vi "Voltage_Sweep_pts.vi"(9 "Vref_Voltage":dbl, 11 "Points":i32) -> (2 "Array":dbl[](array[numeric]))   [LabVIEW 2019]
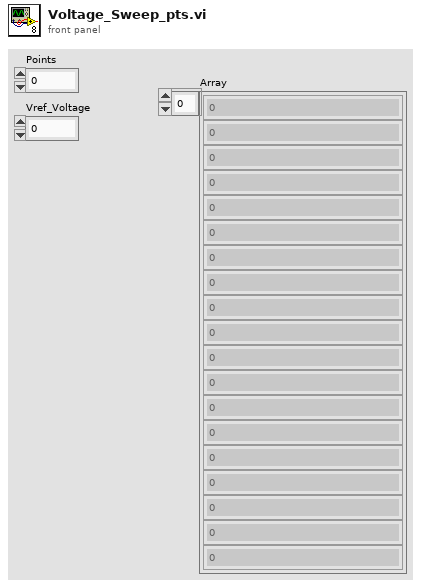
[diagram p1: front panel]
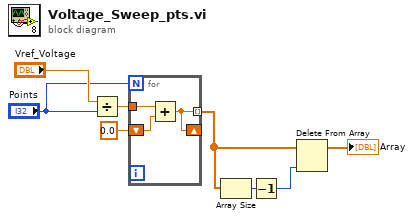
[diagram p0: block diagram]
diagram:
  n1 = Divide(x="Vref_Voltage", y="Points") -> (x/y=w7:dbl)
  n2 = for {
    N: "Points" -> [_]
    shift-right: [w9] -> _
    shift-left: 0.0 -> [w10]
    tunnel: w7 -> [w11]
    tunnel: [w9] -> w4 mode=indexing
    n3 = Add(x=w11, y=w10) -> (x+y=w9:dbl)
  }
  n4 = Array Size(array=w4) -> (size(s)=w2:i32)
  n5 = Decrement(x=w2) -> (x-1=w1:i32)
  n6 = Delete From Array(array=w4, index=w1) -> (array with subset deleted=→"Array":dbl[])  [unwired: 1 in, 1 out]
